vi "OperationsForClick.vi"(9 "Input Coords":T3, 10 "Input Bounds":T1, 11 "Input Position":T2) -> (3 "Clicked Position":i32[](array[numeric]))   [LabVIEW 2019]
uses:
  <vilib>/Utility/miscctls.llb/LVPoint32TypeDef.ctl
  <vilib>/Utility/miscctls.llb/LVPositionTypeDef.ctl
  <vilib>/Utility/miscctls.llb/LVBoundsTypeDef.ctl
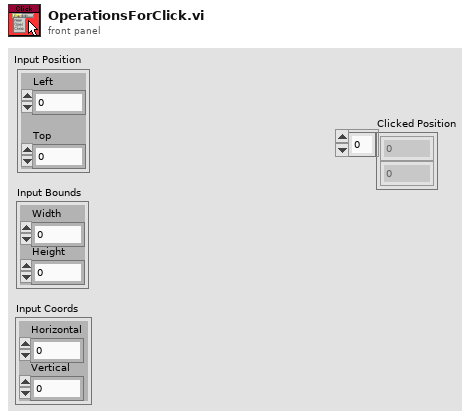
[diagram p1: front panel]
types:
  T1 = typedef "LVBoundsTypeDef.ctl" = cluster{"Width":u32, "Height":u32}
  T2 = typedef "LVPositionTypeDef.ctl" = cluster{"Left":i32, "Top":i32}
  T3 = typedef "LVPoint32TypeDef.ctl" = cluster{"Horizontal":i32, "Vertical":i32}
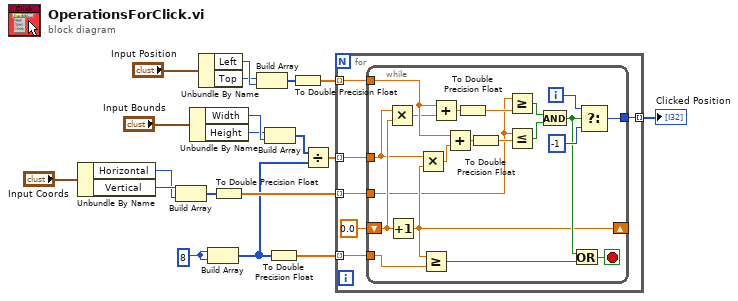
[diagram p0: block diagram]
diagram:
  w3 = 8
  n1 = Unbundle By Name("Input Coords") -> ("Horizontal"=w13:i32, "Vertical"=w14:i32)
  n2 = Build Array(w14, w13) -> (w12:i32[])
  n3 = Unbundle By Name("Input Bounds") -> ("Width"=w7:u32, "Height"=w6:u32)
  n4 = Unbundle By Name("Input Position") -> ("Left"=w5:i32, "Top"=w4:i32)
  n5 = Build Array(w3, w3) -> (w10:i32[])
  n6 = To Double Precision Float(number=w12) -> (double precision float=w17:dbl[])
  n7 = Build Array(w4, w5) -> (w8:i32[])
  n8 = Build Array(w6, w7) -> (w9:u32[])
  n9 = To Double Precision Float(number=w10) -> (double precision float=w16:dbl[])
  n10 = To Double Precision Float(number=w8) -> (double precision float=w15:dbl[])
  n11 = Divide(x=w9, y=w10) -> (x/y=w11:dbl[])
  n12 = for {
    tunnel: w15 -> [w21] mode=indexing
    tunnel: w16 -> [w25] mode=indexing
    tunnel: w11 -> [w22] mode=indexing
    tunnel: w17 -> [w23] mode=indexing
    tunnel: [w20] -> w19 mode=indexing
    n13 = while {
      tunnel: w25 -> [w45]
      tunnel: w23 -> [w26]
      tunnel: w22 -> [w27]
      tunnel: w21 -> [w32]
      tunnel: [w34] -> w20
      shift-right: [w31] -> _
      shift-left: 0.0 -> [w30]
      i -> [w35]
      stop <- w43 stop-if-true
      n14 = Multiply(x=w27, y=w30) -> (x*y=w29:dbl)
      n15 = Increment(x=w30) -> (x+1=w31:dbl)
      n16 = Multiply(x=w27, y=w31) -> (x*y=w28:dbl)
      n17 = Greater Or Equal?(x=w31, y=w45) -> (x >= y?=w44:bool)
      n18 = Add(x=w32, y=w29) -> (x+y=w40:dbl)
      n19 = Add(x=w32, y=w28) -> (x+y=w42:dbl)
      n20 = To Double Precision Float(number=w40) -> (double precision float=w39:dbl)
      n21 = To Double Precision Float(number=w42) -> (double precision float=w41:dbl)
      n22 = Greater Or Equal?(x=w26, y=w39) -> (x >= y?=w38:bool)
      n23 = Less Or Equal?(x=w26, y=w41) -> (x <= y?=w37:bool)
      n24 = And(x=w38, y=w37) -> (x .and. y?=w33:bool)
      n25 = Or(x=w33, y=w44) -> (x .or. y?=w43:bool)
      n26 = Select(t=w35, s=w33, f=-1) -> (s? t:f=w34:i32)
    }
  }
  "Clicked Position" <- w19
